vi "VectorNav recording data state.vi"(4 "next state":T1, 5 "current state":T1, 6 "stop character":u8=44, 7 "input data":u8) -> (0 "state to transition to":T1, 1 "data array length":u8, 2 "recorded data array":u8[](array[numeric]), 3 "Boolean":bool)   [LabVIEW 2009]
uses:
  VectorNav parse QMA state typedef.vi
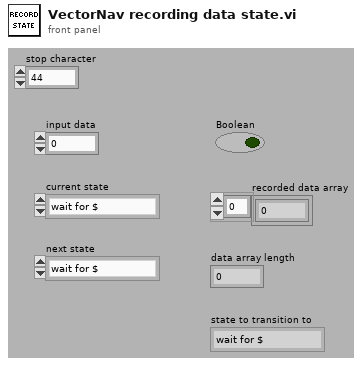
[diagram p1: front panel]
types:
  T1 = typedef "VectorNav parse QMA state typedef.vi" = enum16{"wait for $", "confirm command", "q[0] of quaternion", "q[1] of quaternion", "q[2] of quaternion", "q[3] of quaternion (scalar term)", "X-Axis Magnetic", "Y-Axis Magnetic", "Z-Axis Magnetic", "X-Axis Acceleration", "Y-Axis-Acceleration", "Z-Axis-Acceleration", "Checksum"}
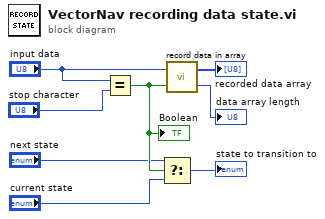
[diagram p0: block diagram]
diagram:
  n1 = Equal?(x="input data", y="stop character") -> (x = y?=w7:bool)
  "Boolean" <- w7
  n2 = Select(t="next state", s=w7, f="current state") -> (s? t:f=→"state to transition to":T1)
  n3 = call "record data in array.vi"("clear data"=w7, "input data"="input data") -> ("data array length"=→"data array length":u8, "recorded data array"=→"recorded data array":u8[])
